vi "Render.vi"(8 "error in (no error)":errorcluster, 11 "XRay Table in":refnum<class "XRay Table.lvclass">=refnum) -> (0 "error out":errorcluster, 2 "Scene Object":refnum<vi>, 3 "XRay Table out":refnum<class "XRay Table.lvclass">)   [LabVIEW 2026, in "XRay Table.lvclass"]
uses:
  XRay Table.lvclass
  XRay Table.lvclass/XRay Table.ctl
  <vilib>/picture/3D Picture Control/Object/Create Object (drawable).vi
  <vilib>/picture/3D Picture Control/Object/Add Object (reference).vi
  <vilib>/picture/3D Picture Control/NI_3D Picture Control.lvlib
panel:
  in  "Translation 3":cluster{"X":sgl, "Y":sgl, "Z":sgl}={"X"=0.0, "Y"=0.0, "Z"=1.0}
  in  "Translation 2":cluster{"X":sgl, "Y":sgl, "Z":sgl}={"X"=0.0, "Y"=0.5, "Z"=0.5}
  in  "Translation":cluster{"X":sgl, "Y":sgl, "Z":sgl}
  in  "Cylinder Radius 3":sgl(slide)=1.0 scale=0.1..2.0
  in  "Cylinder Height 3":sgl(slide)=2.0 scale=0.1..5.0
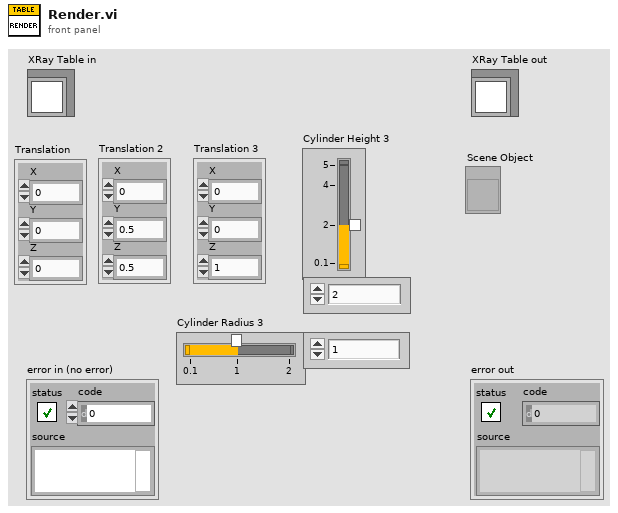
[diagram p1: front panel]
types:
  T1 = enum16{"Inherit Value", "Points", "Wireframe", "Polygons"}
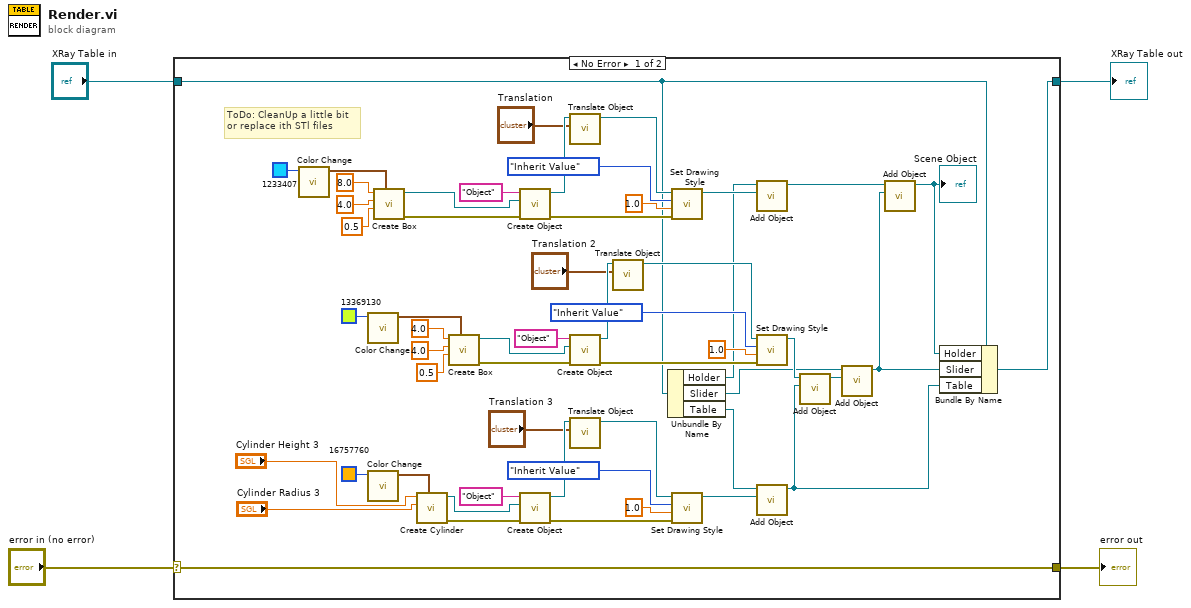
[diagram p0: block diagram]
diagram:
  n1 = case shown="No Error" "error in (no error)" {
    selector: "error in (no error)" -> [w59 w61]
    tunnel: [w59 w61] -> w3
    tunnel: [w20 w60] -> w1
    tunnel: "XRay Table in" -> [w19 w60]
    frame No Error {
      # "ToDo: CleanUp a little bit\nor replace ith STl files"
      n2 = call <vilib>:"Color Change.vi"("Color"=u32 1233407) -> ("RGBA"=w47:cluster{"R":sgl, "G":sgl, "B":sgl, "A":sgl})  [unwired: 10 in]
      n3 = call <vilib>:"Color Change.vi"("Color"=u32 13369130) -> ("RGBA"=w44:cluster{"R":sgl, "G":sgl, "B":sgl, "A":sgl})  [unwired: 10 in]
      n4 = call <vilib>:"Color Change.vi"("Color"=u32 16757760) -> ("RGBA"=w23:cluster{"R":sgl, "G":sgl, "B":sgl, "A":sgl})  [unwired: 10 in]
      n5 = call <vilib>:"Create Box.vi"("Color"=w47, "Length Z"=sgl 0.5 ("Box Length Z 4"), "Length Y"=sgl 4.0 ("Box Length Y 4"), "Length X"=sgl 8.0 ("Box Length X 4")) -> ("error out"=w49:errorcluster, "New Box Refnum"=w53:refnum<vi>)  [unwired: 6 in]
      n6 = call <vilib>:"Create Cylinder.vi"("Color"=w23, "Radius"="Cylinder Radius 3", "Height"="Cylinder Height 3") -> ("error out"=w21:errorcluster, "New Cylinder Refnum"=w22:refnum<vi>)  [unwired: 7 in]
      n7 = call <vilib>:"Create Box.vi"("Color"=w44, "Length Z"=sgl 0.5 ("Box Length Z 4"), "Length Y"=sgl 4.0 ("Box Length Y 4"), "Length X"=sgl 4.0 ("Box Length X 4")) -> ("error out"=w42:errorcluster, "New Box Refnum"=w38:refnum<vi>)  [unwired: 6 in]
      n8 = call-poly <vilib>:"Create Object.vi"("error in (no error)"=w49, "Geometry"=w53, "Name"="Object") -> ("error out"=w52:errorcluster, "Scene:New Object"=w54:refnum<vi>)  [unwired: 7 in]
      n9 = call-poly <vilib>:"Create Object.vi"("error in (no error)"=w21, "Geometry"=w22, "Name"="Object") -> ("error out"=w28:errorcluster, "Scene:New Object"=w29:refnum<vi>)  [unwired: 7 in]
      n10 = call <vilib>:"Translate Object.vi"("Translation"="Translation", "Scene.Object In"=w54) -> ("Scene.Object Out"=w55:refnum<vi>)  [unwired: 8 in, 1 out]
      n11 = call-poly <vilib>:"Create Object.vi"("error in (no error)"=w42, "Geometry"=w38, "Name"="Object") -> ("error out"=w39:errorcluster, "Scene:New Object"=w37:refnum<vi>)  [unwired: 7 in]
      n12 = call <vilib>:"Translate Object.vi"("Translation"="Translation 3", "Scene.Object In"=w29) -> ("Scene.Object Out"=w30:refnum<vi>)  [unwired: 8 in, 1 out]
      n13 = call <vilib>:"Translate Object.vi"("Translation"="Translation 2", "Scene.Object In"=w37) -> ("Scene.Object Out"=w36:refnum<vi>)  [unwired: 8 in, 1 out]
      n14 = Unbundle By Name(w19) -> ("Holder"=w7:refnum<vi>, "Slider"=w10:refnum<vi>, "Table"=w14:refnum<vi>)
      n15 = call <vilib>:"Set Drawing Style.vi"("error in (no error)"=w52, "Size"=1.0, "Mode"=T1."Inherit Value" ("Draw Mode"), "Scene Object In"=w55) -> ("Scene Object Out"=w15:refnum<vi>)  [unwired: 6 in, 1 out]
      n16 = call <vilib>:"Set Drawing Style.vi"("error in (no error)"=w28, "Size"=1.0, "Mode"=T1."Inherit Value" ("Draw Mode"), "Scene Object In"=w30) -> ("Scene Object Out"=w13:refnum<vi>)  [unwired: 6 in, 1 out]
      n17 = call-poly <vilib>:"Add Object.vi"("New Object In"=w15, "Scene Object In"=w7) -> ("Scene Object Out"=w6:refnum<vi>)  [unwired: 7 in, 2 out]
      n18 = call <vilib>:"Set Drawing Style.vi"("error in (no error)"=w39, "Size"=1.0, "Mode"=T1."Inherit Value" ("Draw Mode"), "Scene Object In"=w36) -> ("Scene Object Out"=w12:refnum<vi>)  [unwired: 6 in, 1 out]
      n19 = call-poly <vilib>:"Add Object.vi"("New Object In"=w13, "Scene Object In"=w14) -> ("Scene Object Out"=w11:refnum<vi>)  [unwired: 7 in, 2 out]
      n20 = call-poly <vilib>:"Add Object.vi"("New Object In"=w11, "Scene Object In"=w12) -> ("Scene Object Out"=w9:refnum<vi>)  [unwired: 7 in, 2 out]
      n21 = call-poly <vilib>:"Add Object.vi"("New Object In"=w9, "Scene Object In"=w10) -> ("Scene Object Out"=w8:refnum<vi>)  [unwired: 7 in, 2 out]
      n22 = call-poly <vilib>:"Add Object.vi"("New Object In"=w8, "Scene Object In"=w6) -> ("Scene Object Out"=w5:refnum<vi>)  [unwired: 7 in, 2 out]
      "Scene Object" <- w5
      n23 = Bundle By Name(cluster=w19, "Holder"=w5, "Slider"=w8, "Table"=w11) -> (w20:refnum<class "XRay Table.lvclass">)
    }
    frame Error {
    }
  }
  "error out" <- w3
  "XRay Table out" <- w1
